vi "PH_TKTDS-30xx.Configure Channel.vi"(0 "i ref in":refnum<vi>, 1 "GUI Element Name":string="N/A", 2 "Channel Configuration":T1={"Channel Name"="CH1", "Input Impedance"="MEG", "Max Input Frequency"="TWENTY", "Vertical Coupling"=1, "Channel Enabled"=TRUE, "Probe Attenuation"=1.0, "Vertical Range"=100.0, "Vertical Offset"=0.0} {"Vertical Offset" format="%#_6p"; "Vertical Range" items=["1mV"=0.001, "2mV"=0.002, "5mV"=0.005, "10mV"=0.01, "20mV"=0.02, "50mV"=0.05, "100mV"=0.1, "200mV"=0.2, "500mV"=0.5, "1V"=1.0]; "Probe Attenuation" format="%#.2f"}, 5 "error IO":errorcluster) -> (14 "i ref out":refnum<vi>, 19 "error out":errorcluster)   [LabVIEW 2014, in "PH_TKTDS-30xx.lvlib"]
doc: "If the connection is established, the channel configuration is set and written to own attributes as well as the errors."
uses:
  PH_TKTDS-30xx.lvlib
  PH_TKTDS-30xx.Channel Config.ctl
  instr.lib/TKDS3032-PHELIX/tktds3032-PHELIX - Driver np.lvlib
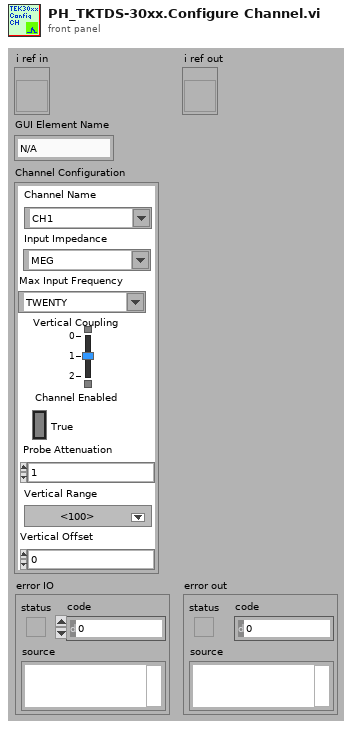
[diagram p1: front panel]
types:
  T1 = typedef "PH_TKTDS-30xx.lvlib/PH_TKTDS-30xx.Channel Config.ctl" = cluster{"Channel Name":string, "Input Impedance":string, "Max Input Frequency":string, "Vertical Coupling":i32, "Channel Enabled":bool, "Probe Attenuation":dbl, "Vertical Range":dbl, "Vertical Offset":dbl}
  T2 = typedef "PH_TKTDS-30xx.lvlib/PH_TKTDS-30xx.i attribute.ctl" = cluster{"Default VISA Resource":string, "VISA Resource Name":refnum<visa-resource-name>, "Revision":cluster{"Instrument Driver":string, "Instrument Firmware":string}, "Selftest":cluster{"Result":u32, "Message":string}, "Channels":T1[], "Trigger Configuration":T3, "Acquisition Configuration":T4, "Fetched Waveforms":T5[], "GUI Refs":T6, "GUI Refs Channels":refnum<vi>[], "State":T7, "Error Message":string, "Allow Prdc Loop?":bool}
  T3 = typedef "PH_TKTDS-30xx.lvlib/PH_TKTDS-30xx.Trigger Config.ctl" = cluster{"Source":string, "Slope":i32, "Level [V]":dbl}
  T4 = typedef "PH_TKTDS-30xx.lvlib/PH_TKTDS-30xx.Acquisition Config.ctl" = cluster{"Time base":dbl, "Record Length":u16, "Start Time":dbl, "Type":i32, "Continuous":bool}
  T5 = typedef "PH_TKTDS-30xx.lvlib/PH_TKTDS-30xx.fetched Waveform.ctl" = cluster{"Source":string, "Actual Points":u32, "Initial X":dbl, "X Increment":dbl, "Waveform Array":dbl[]}
  T6 = typedef "PH_TKTDS-30xx.lvlib/PH_TKTDS-30xx.GUI Refs.ctl" = cluster{"Trigger":refnum<vi>, "Acquisition":refnum<vi>, "Graph":refnum<vi>, "State":refnum<vi>, "Delete":refnum<vi>, "Channel to be positioned":refnum<vi>, "Postion":refnum<vi>, "Display Intensity":refnum<vi>, "VISA Resource":refnum<vi>}
  T7 = typedef "PH_StatusHandler.lvlib/PH_StatusHandler.Status.ctl" = i16
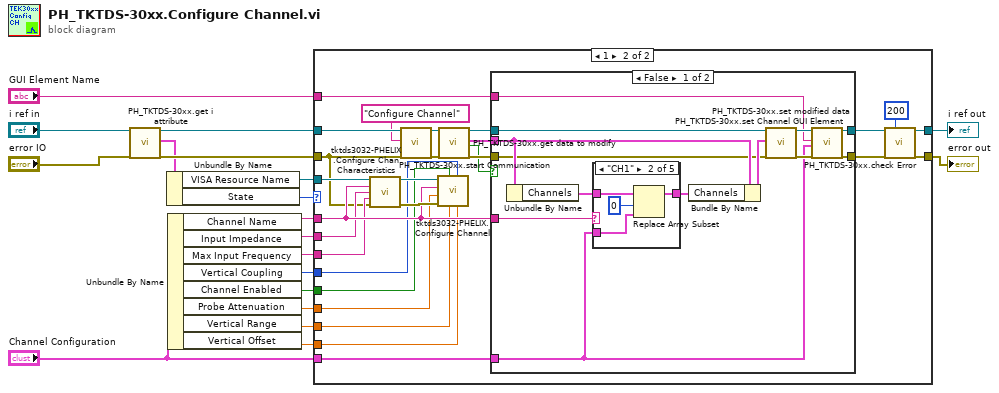
[diagram p0: block diagram]
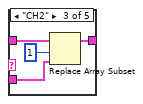
[diagram p4: hidden frame]
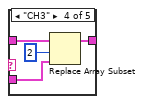
[diagram p5: hidden frame]
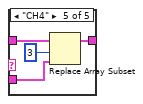
[diagram p6: hidden frame]
diagram:
  n1 = call "PH_TKTDS-30xx.get i attribute.vi"("i ref in"="i ref in", "error in (no error)"="error IO") -> ("i ref out"=w14:refnum<vi>, "i attribute"=w16:T2, "error out"=w18:errorcluster)  [unwired: 15 in]
  n2 = Unbundle By Name(w16) -> ("VISA Resource Name"=w17:refnum<visa-resource-name>, "State"=w3:T7)
  n3 = Unbundle By Name("Channel Configuration") -> ("Channel Name"=w11:string, "Input Impedance"=w10:string, "Max Input Frequency"=w9:string, "Vertical Coupling"=w8:i32, "Channel Enabled"=w7:bool, "Probe Attenuation"=w6:dbl, "Vertical Range"=w5:dbl, "Vertical Offset"=w4:dbl)
  n4 = case shown="1" w3 {
    tunnel: w14 -> [w21 w48]
    tunnel: w17 -> [_ w42]
    tunnel: [w20 w28] -> w12
    tunnel: w18 -> [w20 w27]
    tunnel: [w21 w24] -> w19
    tunnel: w11 -> [_ w39]
    tunnel: w10 -> [_ w38]
    tunnel: w9 -> [_ w37]
    tunnel: w7 -> [_ w36]
    tunnel: w8 -> [_ w35]
    tunnel: w6 -> [_ w34]
    tunnel: w5 -> [_ w33]
    tunnel: w4 -> [_ w32]
    tunnel: "Channel Configuration" -> [_ w31]
    tunnel: "GUI Element Name" -> [_ w30]
    frame Default {
    }
    frame 1 {
      n5 = call "tktds3032-PHELIX.Configure Chan Characteristics.vi"("VISA Resource Name"=w42, "Channel Name (\"CH1\")"=w39, "Input Impedance (1.0 mega ohm)"=w38, "Max Input Frequency (20.0E+6 Hz)"=w37, "error in (no error)"=w27) -> ("VISA Resource Name Out"=w41:refnum<visa-resource-name>, "error out"=w40:errorcluster)  [unwired: 9 in]
      n6 = call "PH_TKTDS-30xx.start Communication.vi"("i ref in"=w48, "Action"="Configure Channel", "error in"=w27) -> ("i ref out"=w29:refnum<vi>, "error out"=w26:errorcluster)  [unwired: 15 in]
      n7 = call "tktds3032-PHELIX.Configure Channel.vi"("Vertical Offset (0.0 V)"=w32, "Vertical Coupling (DC)"=w35, "Vertical Range"=w33, "Channel Enabled (True)"=w36, "error in (no error)"=w40, "Probe Attenuation (1.0)"=w34, "Channel Name (\"CH1\")"=w39, "VISA Resource Name"=w41) -> ()  [unwired: 2 in, 2 out]
      n8 = call "PH_TKTDS-30xx.get data to modify.vi"("i ref in"=w29, "error in (no error)"=w26) -> ("i ref out"=w45:refnum<vi>, "i attribute"=w43:T2, "timed out"=w44:bool, "error out"=w46:errorcluster)  [unwired: 14 in]
      n9 = case shown="False" w44 {
        tunnel: [w51 w79] -> w47
        tunnel: w46 -> [w55 w79]
        tunnel: w45 -> [w61 w80]
        tunnel: [w53 w80] -> w25
        tunnel: w43 -> [w56 _]
        tunnel: w39 -> [w59 _]
        tunnel: w31 -> [w49 _]
        tunnel: w30 -> [w50 _]
        frame False {
          n10 = Unbundle By Name(w56) -> ("Channels"=w57:T1[])
          n11 = case shown="\"CH1\"" w59 {
            tunnel: [w62 w65 w69 w73 w77] -> w58
            tunnel: w57 -> [w62 w66 w70 w74 w78]
            tunnel: w49 -> [_ w63 w67 w71 w75]
            frame Default {
            }
            frame "CH1" {
              n12 = Replace Array Subset(array=w66, new element=w63, index=0) -> (w65:T1[])
            }
            frame "CH2" {
              n13 = Replace Array Subset(array=w70, new element=w67, index=1) -> (w69:T1[])
            }
            frame "CH3" {
              n14 = Replace Array Subset(array=w74, new element=w71, index=2) -> (w73:T1[])
            }
            frame "CH4" {
              n15 = Replace Array Subset(array=w78, new element=w75, index=3) -> (w77:T1[])
            }
          }
          n16 = Bundle By Name(cluster=w56, "Channels"=w58) -> (w60:T2)
          n17 = call "PH_TKTDS-30xx.set modified data.vi"("i ref in"=w61, "i attribute"=w60, "error in (no error)"=w55) -> ("i ref out"=w54:refnum<vi>, "error out"=w52:errorcluster)  [unwired: 15 in]
          n18 = call "PH_TKTDS-30xx.set Channel GUI Element.vi"("i ref in"=w54, "GUI Element Name"=w50, "Channel Config"=w49, "error in"=w52) -> ("i ref out"=w53:refnum<vi>, "error out"=w51:errorcluster)  [unwired: 14 in]
        }
        frame True {
        }
      }
      n19 = call "PH_TKTDS-30xx.check Error.vi"("i ref in"=w25, "Waiting Time [ms]"=u32 200, "error in"=w47) -> ("i ref out"=w24:refnum<vi>, "error out"=w28:errorcluster)  [unwired: 15 in]
    }
  }
  "i ref out" <- w19
  "error out" <- w12
